vi "BRig_RT__Case_Idle__State_Idle__getAudioParam.vi"(10 "input_dataExp":u16[](array[numeric]), 11 "input_dataMTrig":u16[](array[numeric])) -> (0 "output_Audio_freq_R":u8, 1 "output_Audio_amp_R":u16, 2 "output_Audio_freq_L":u8, 3 "output_Audio_amp_L":u16, 5 "output_state":T1)   [LabVIEW 2014]
uses:
  myRIO_BRig_RT__Case_NonExp_stateList.ctl
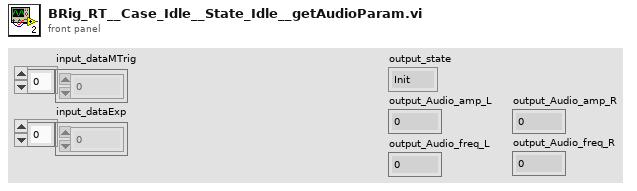
[diagram p1: front panel]
types:
  T1 = typedef "myRIO_BRig_RT__Case_NonExp_stateList.ctl" = enum16{"Init", "UploadSettings_pre", "UploadSettings_Read_dataExp", "UploadSettings_dataExp_1", "UploadSettings_dataExp_2", "UploadSettings_Read_dataLC", "UploadSettings_dataLC_1", "UploadSettings_dataLC_2", "UploadSettings_dataLC_3", "UploadSettings_dataLC_4", "UploadSettings_Read_dataMTrig", "UploadSettings_dataMTrig_1", "UploadSettings_post", "Idle_pre", "IdleEmpty", "IdleEmpty2", "IdleEmpty3", "IdleEmpty4", "Idle", "Idle_2", "Idle_3", "Idle_4", "Idle_5", "Idle_6", "Idle_post", "Cue_pre__pre", "Cue_pre", "Cue", "Cue_LED", "Cue_post", "RewardCalibration_pre", "RewardCalibration", "DispenseWater_pre__pre", "DispenseWater_pre", "DispenseWater", "DispenseWater_post", "TestConnection", "SendData", "Get_FPGA_count_per_ms", "End", "commTCP_connect"}
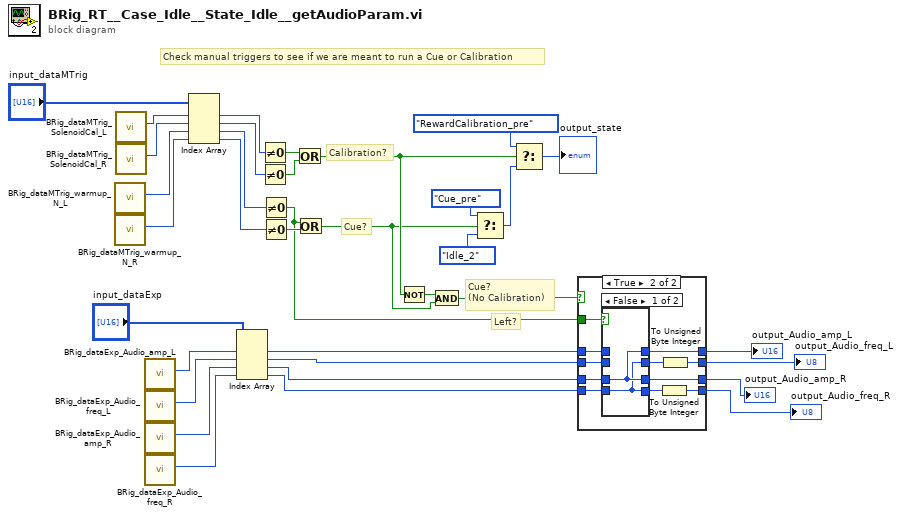
[diagram p0: block diagram]
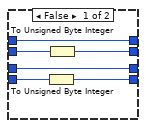
[diagram p2: hidden frame]
diagram:
  # "Left?"
  # "Cue?\n(No Calibration)"
  # "Cue?"
  # "Calibration?"
  # "Check manual triggers to see if we are meant to run a Cue or Calibration"
  n1 = call "BRig_dataMTrig_warmup_N_L.vi"() -> ("output_warmup_N_L"=w23:i32)  [unwired: 11 in]
  n2 = call "BRig_dataMTrig_warmup_N_R.vi"() -> ("output_warmup_N_R"=w22:i32)  [unwired: 11 in]
  n3 = call "BRig_dataMTrig_SolenoidCal_L.vi"() -> ("output_SolenoidCal_L"=w30:i32)  [unwired: 11 in]
  n4 = call "BRig_dataMTrig_SolenoidCal_R.vi"() -> ("output_SolenoidCal_R"=w29:i32)  [unwired: 11 in]
  n5 = call "BRig_dataExp_Audio_amp_L.vi"() -> ("output_Audio_amp__L"=w34:i32)  [unwired: 11 in]
  n6 = call "BRig_dataExp_Audio_freq_L.vi"() -> ("output_Audio_freq__L"=w33:i32)  [unwired: 11 in]
  n7 = call "BRig_dataExp_Audio_amp_R.vi"() -> ("output_Audio_amp__R"=w32:i32)  [unwired: 11 in]
  n8 = call "BRig_dataExp_Audio_freq_R.vi"() -> ("output_Audio_freq__R"=w31:i32)  [unwired: 11 in]
  n9 = Index Array(array="input_dataMTrig", index #1=w30, index #2=w29, index #3=w23, index #4=w22) -> (element #1=w28:u16, element #2=w27:u16, element #3=w21:u16, element #4=w20:u16)
  n10 = Index Array(array="input_dataExp", index #1=w34, index #2=w33, index #3=w32, index #4=w31) -> (element #1=w15:u16, element #2=w14:u16, element #3=w13:u16, element #4=w12:u16)
  n11 = Not Equal To 0?(x=w28) -> (x != 0?=w25:bool)
  n12 = Not Equal To 0?(x=w27) -> (x != 0?=w26:bool)
  n13 = Not Equal To 0?(x=w21) -> (x != 0?=w6:bool)
  n14 = Not Equal To 0?(x=w20) -> (x != 0?=w7:bool)
  n15 = Or(x=w25, y=w26) -> (x .or. y?=w11:bool)
  n16 = Or(x=w6, y=w7) -> (x .or. y?=w9:bool)
  n17 = Not(x=w11) -> (.not. x?=w10:bool)
  n18 = And(x=w10, y=w9) -> (x .and. y?=w8:bool)
  n19 = Select(t=myRIO_BRig_RT__Case_NonExp_stateList."Cue_pre" ("Enum"), s=w9, f=myRIO_BRig_RT__Case_NonExp_stateList."Idle_2" ("Enum")) -> (s? t:f=w17:T1)
  n20 = Select(t=myRIO_BRig_RT__Case_NonExp_stateList."RewardCalibration_pre" ("Enum"), s=w11, f=w17) -> (s? t:f=→"output_state":T1)
  n21 = case shown="True" w8 {
    tunnel: w15 -> [w39 w51]
    tunnel: w14 -> [w41 w50]
    tunnel: w13 -> [w37 w49]
    tunnel: w12 -> [w40 w48]
    tunnel: [w39 w43] -> w4
    tunnel: [w38 w42] -> w3
    tunnel: [w37 w44] -> w2
    tunnel: [w36 w45] -> w1
    tunnel: w6 -> [_ w52]
    frame False {
      n22 = To Unsigned Byte Integer(number=w40) -> (unsigned 8bit integer=w36:u8)
      n23 = To Unsigned Byte Integer(number=w41) -> (unsigned 8bit integer=w38:u8)
    }
    frame True {
      n24 = case shown="False" w52 {
        tunnel: w51 -> [_ w56]
        tunnel: w50 -> [_ w55]
        tunnel: w49 -> [w54 _]
        tunnel: w48 -> [w53 _]
        tunnel: [w54 w56] -> w43
        tunnel: [w53 w55] -> w47
        tunnel: [w54 w56] -> w44
        tunnel: [w53 w55] -> w46
        frame False {
        }
        frame True {
        }
      }
      n25 = To Unsigned Byte Integer(number=w46) -> (unsigned 8bit integer=w45:u8)
      n26 = To Unsigned Byte Integer(number=w47) -> (unsigned 8bit integer=w42:u8)
    }
  }
  "output_Audio_amp_L" <- w4
  "output_Audio_freq_L" <- w3
  "output_Audio_amp_R" <- w2
  "output_Audio_freq_R" <- w1
